vi "Start Module.vi"(6 "Show Main VI Diagram on Init (F)":bool, 8 "error in":errorcluster) -> (0 "error out":errorcluster, 1 "Wait for Event Sync?":bool, 2 "CML UI Broadcast Events":T1, 3 "Module Was Already Running?":bool)   [LabVIEW 2024, in "CML UI.lvlib"]
doc: "Launches the Module Main.vi.\n_____\nBased on DQMH Project Template 4.0.0.47.\n\n<b>Note:</b> This VI was modified by the <b>Validate DQMH Module</b> tool to add calls to the Semaphore VIs to synchronize actions between the Start Module and Stop Module VIs.\n_____\nBased on DQMH Project Template 7.0.1.1316."
uses:
  CML UI.lvlib
  Broadcast Events--cluster.ctl
  Did Init Argument--cluster.ctl
  Status Updated Argument--cluster.ctl
  Error Reported Argument--cluster.ctl
  Stop Argument--cluster.ctl
  Get Module Execution Status Argument--cluster.ctl
  <vilib>/Delacor/Delacor QMH/Libraries/Module Admin_class/Delacor_lib_QMH_Module Admin.lvclass
  <vilib>/Delacor/Delacor QMH/Libraries/Module Admin_class/Delacor_lib_QMH_Module Admin.lvclass/Delacor_lib_QMH_Module Admin.ctl
  <vilib>/Delacor/Delacor QMH/Libraries/Module Admin_class/Delacor_lib_QMH_Set External Launch.vi
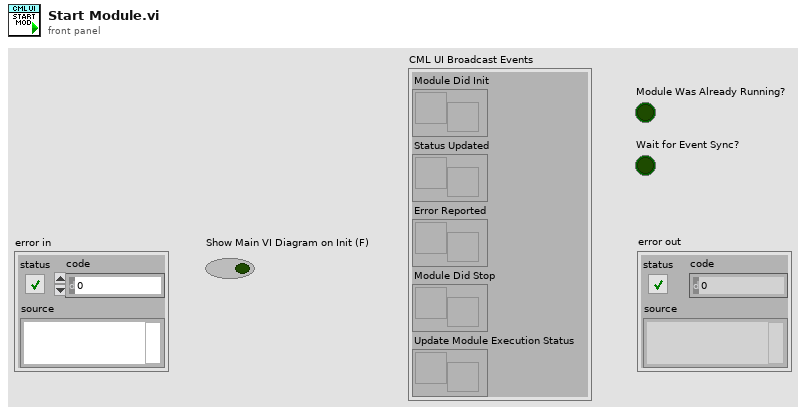
[diagram p1: front panel]
types:
  T1 = typedef "CML UI.lvlib/Broadcast Events--cluster.ctl" = cluster{"Module Did Init":refnum<user-event>, "Status Updated":refnum<user-event>, "Error Reported":refnum<user-event>, "Module Did Stop":refnum<user-event>, "Update Module Execution Status":refnum<user-event>}
  T2 = enum32{"Bad", "Idle", "Run top level", "Running"}
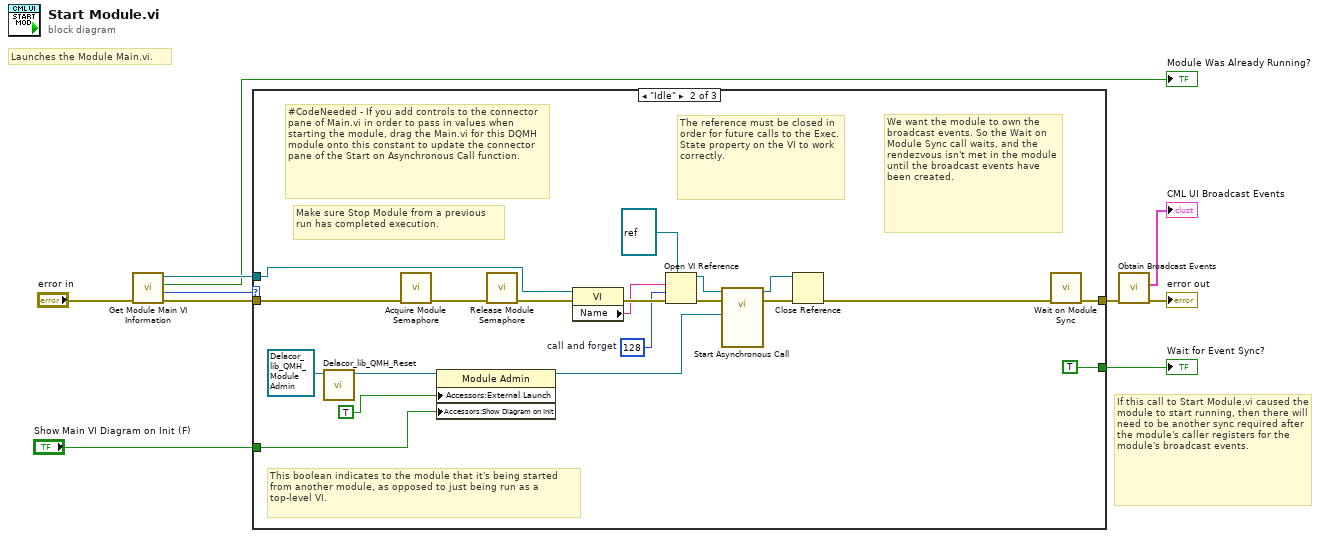
[diagram p0: block diagram]
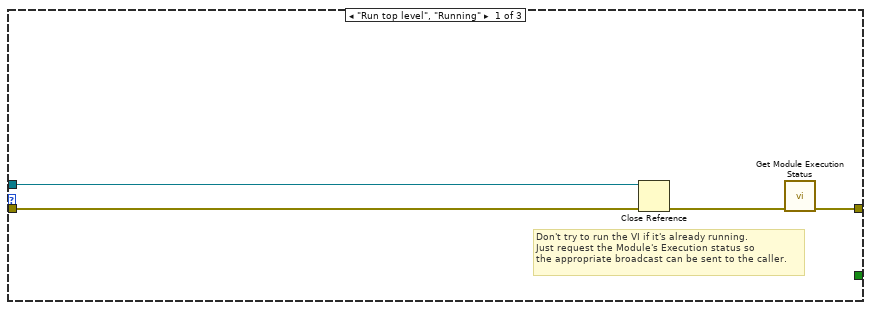
[diagram p2: hidden frame]
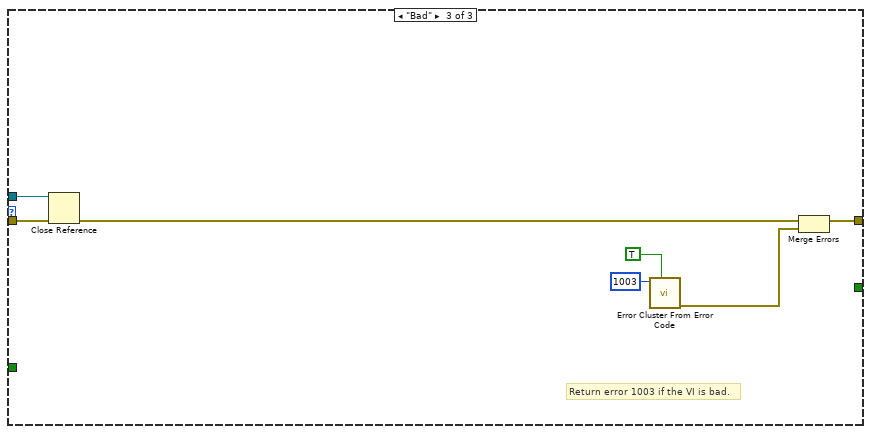
[diagram p3: hidden frame]
diagram:
  # "If this call to Start Module.vi caused the module to start running, then there will need to be another sync required after the module's caller registers for the module's broadcast events."
  # "Launches the Module Main.vi."
  n1 = call "Get Module Main VI Information.vi"("error in"="error in") -> ("error out"=w9:errorcluster, "Execution State"=w4:T2, "Is Module Running?"=→"Module Was Already Running?":bool, "Module Main VI"=w8:refnum<vi>)  [unwired: 7 in]
  n2 = case shown="\"Idle\"" w4 {
    tunnel: w9 -> [w14 w22 w41]
    tunnel: w8 -> [w13 w19 w40]
    tunnel: [w11 w34 w38] -> w7
    tunnel: [_ TRUE _] -> w5
    tunnel: "Show Main VI Diagram on Init (F)" -> [_ w15 _]
    frame "Run top level", "Running" {
      # "Don't try to run the VI if it's already running.\nJust request the Module's Execution status so\nthe appropriate broadcast can be sent to the caller."
      n3 = Close Reference(reference=w13, error in (no error)=w14) -> (error out=w12:errorcluster)
      n4 = call "Get Module Execution Status.vi"("error in"=w12) -> ("error out"=w11:errorcluster)  [unwired: 10 in]
    }
    frame "Idle" {
      w28 = 128  # call and forget
      # "Make sure Stop Module from a previous run has completed execution."
      # "#CodeNeeded - If you add controls to the connector pane of Main.vi in order to pass in values when starting the module, drag the Main.vi for this DQMH module onto this constant to update the connector pane of the Start on Asynchronous Call function."
      # "The reference must be closed in order for future calls to the Exec.State property on the VI to work correctly."
      # "We want the module to own the broadcast events. So the Wait on Module Sync call waits, and the rendezvous isn't met in the module until the broadcast events have been created."
      # "This boolean indicates to the module that it's being started from another module, as opposed to just being run as a top-level VI."
      n5 = call-dynamic "Delacor_lib_QMH_Reset.vi"("Mod Admin in"=refnum<class "Delacor_lib_QMH_Module Admin.lvclass"> refnum) -> ("Mod Admin out"=w32:refnum<class "Delacor_lib_QMH_Module Admin.lvclass">)  [unwired: 9 in, 1 out]
      n6 = call "Acquire Module Semaphore.vi"("error in"=w22) -> ("error out"=w17:errorcluster)  [unwired: 10 in]
      n7 = property on="Property Node" class="Module Admin"(reference=w32, "Accessors:External Launch"=TRUE, "Accessors:Show Diagram on Init"=w15) -> (reference out=w20:refnum<class "Delacor_lib_QMH_Module Admin.lvclass">)  [unwired: 1 in, 1 out]
      n8 = call "Release Module Semaphore.vi"("error in"=w17) -> ("error out"=w16:errorcluster)  [unwired: 10 in]
      n9 = property class="VI"(reference=w19, error in=w16) -> (error out=w29:errorcluster, "Name"=w23:string)  [unwired: 1 out]
      n10 = Open VI Reference(type specifier VI Refnum (for type only)=refnum<vi> refnum, vi path=w23, options=w28, error in (no error)=w29) -> (vi reference=w26:refnum<vi>, error out=w27:errorcluster)  [unwired: 2 in]
      n11 = call-by-ref "Start Asynchronous Call"(reference=w26, error in=w27, "Module Admin"=w20) -> (reference out=w24:refnum<vi>, error out=w25:errorcluster)  [unwired: 11 in]
      n12 = Close Reference(reference=w24, error in (no error)=w25) -> (error out=w21:errorcluster)
      n13 = call "Wait on Module Sync.vi"("error in"=w21) -> ("error out"=w34:errorcluster)  [unwired: 10 in]
    }
    frame "Bad" {
      # "Return error 1003 if the VI is bad."
      n14 = Close Reference(reference=w40, error in (no error)=w41) -> (error out=w39:errorcluster)
      n15 = call <vilib>:"Error Cluster From Error Code.vi"("show call chain? (False)"=TRUE, "error code (0)"=1003) -> ("error out"=w37:errorcluster)  [unwired: 7 in]
      n16 = Merge Errors(w39, w37) -> (w38:errorcluster)
    }
  }
  "Wait for Event Sync?" <- w5
  n17 = call "Obtain Broadcast Events.vi"("error in"=w7) -> ("error out"=→"error out":errorcluster, "CML UI Broadcast Events"=→"CML UI Broadcast Events":T1)  [unwired: 9 in]
